vi "4_ClearQueue.vi"(8 "error in (no error)":errorcluster caption="错误输入（无错误）", 10 "QueueName":T1, 11 "Queue In":refnum<queue>[](array[refnum])) -> (0 "error out":errorcluster caption="错误输出", 3 "Queue Out":refnum<queue>[](array[refnum]))   [LabVIEW 2017]
uses:
  Ctrls/QueueDataForm.ctl
  Ctrls/QueueName.ctl
panel:
  # "Stop"
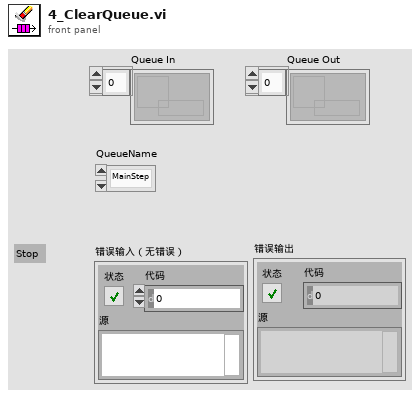
[diagram p1: front panel]
types:
  T1 = typedef "QueueName.ctl" = enum16{"MainStep", "AutoRun", "胶高"}
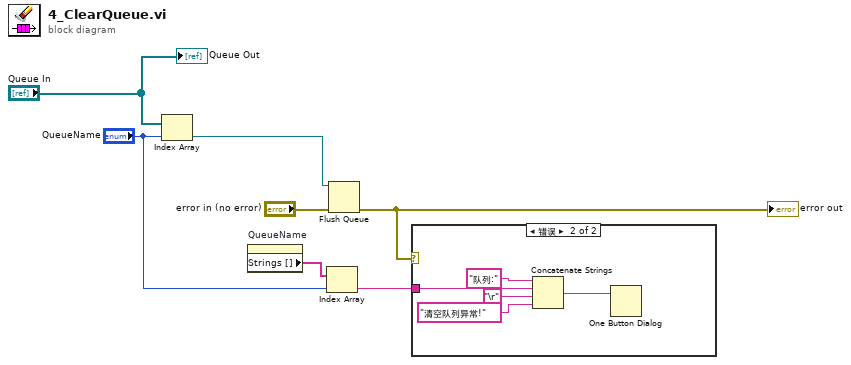
[diagram p0: block diagram]
diagram:
  n1 = Index Array(array="Queue In", index="QueueName") -> (element=w6:refnum<queue>)
  n2 = property on="QueueName" class="Enum (严格)"() -> ("Strings []"=w3:string[])  [unwired: 2 in, 2 out]
  n3 = Index Array(array=w3, index="QueueName") -> (element=w1:string)
  n4 = Flush Queue(queue=w6, error in (no error)="error in (no error)") -> (error out=w4:errorcluster)  [unwired: 2 out]
  "error out" <- w4
  n5 = case shown="错误" w4 {
    tunnel: w1 -> [_ w11]
    frame No Error {
    }
    frame Error {
      n6 = Concatenate Strings("队列:", w11, "\r", "清空队列异常!" ("字符串")) -> (w8:string)
      n7 = One Button Dialog(message=w8) -> ()  [unwired: 1 in, 1 out]
    }
  }
  "Queue Out" <- "Queue In"
